vi "singleStamp.vi"() -> ()   [LabVIEW 2017]
uses:
  Gantry/Shared Components/Gantry Class/Type Definitions/Virtual Modes.ctl
  Gantry/Shared Components/Gantry Class/Gantry.lvclass
  Gantry/Shared Components/FlexWorktable/FlexWorktable.lvclass
panel:
  out "error out":errorcluster
  in  "Config Folder":path=path "C:/Users/husker/Desktop/gantry/Config"
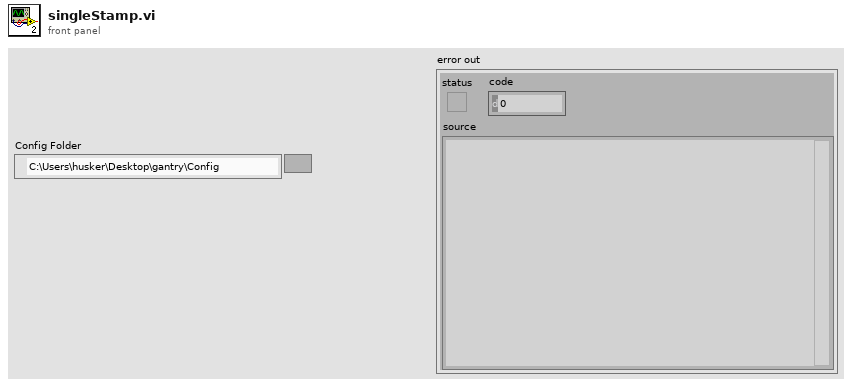
[diagram p1: front panel]
types:
  T1 = typedef "Virtual Modes.ctl" = enum16{"Nonvirtual", "Virtual"}
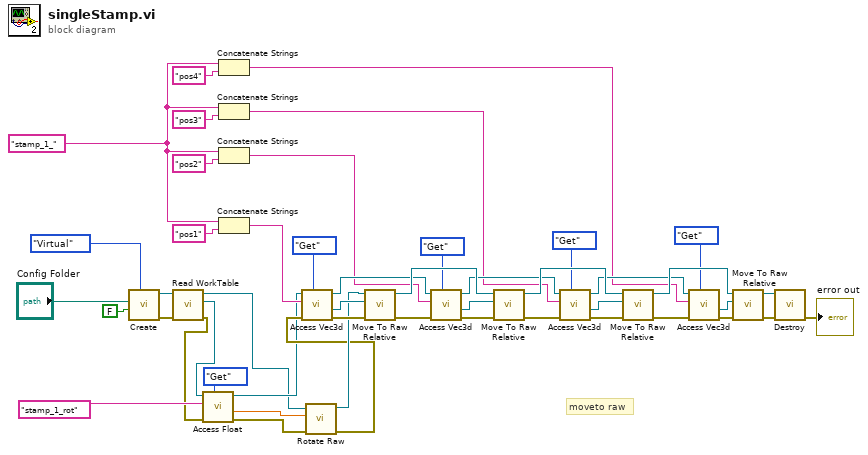
[diagram p0: block diagram]
diagram:
  w17 = "stamp_1_"
  # "moveto raw"
  n1 = call "Create.vi"("Virtual Mode"=Virtual_Modes."Virtual", "HOME?"=FALSE, "Config Folder"="Config Folder") -> ("error out"=w43:errorcluster, "Gantry out"=w44:refnum<class "Gantry.lvclass">)  [unwired: 6 in, 1 out]
  n2 = call-dynamic "Read WorkTable.vi"("error in"=w43, "Gantry Class in"=w44) -> ("error out"=w8:errorcluster, "Worktable"=w9:refnum<class "FlexWorktable.lvclass">, "Gantry Class out"=w2:refnum<class "Gantry.lvclass">)  [unwired: 7 in]
  n3 = call-dynamic "Access Float.vi"("Get/Set"=enum16{"Get", "Set"}."Get", "error in (no error)"=w8, "Key"="stamp_1_rot", "FlexWorktable in"=w9) -> ("error out"=w6:errorcluster, "Value out"=w4:dbl, "FlexWorktable out"=w3:refnum<class "FlexWorktable.lvclass">)  [unwired: 5 in]
  n4 = Concatenate Strings(w17, "pos4" ("string")) -> (w21:string)
  n5 = Concatenate Strings(w17, "pos3" ("string")) -> (w23:string)
  n6 = Concatenate Strings(w17, "pos2" ("string")) -> (w24:string)
  n7 = Concatenate Strings(w17, "pos1" ("string")) -> (w19:string)
  n8 = call-dynamic "Rotate Raw.vi"("error in"=w6, "position(deg)"=w4, "Gantry in"=w2) -> ("error out"=w5:errorcluster, "Gantry out"=w7:refnum<class "Gantry.lvclass">)  [unwired: 7 in]
  n9 = call-dynamic "Access Vec3d.vi"("Get/Set"=enum16{"Get", "Set"}."Get", "error in (no error)"=w5, "Key"=w19, "FlexWorktable in"=w3) -> ("error out"=w14:errorcluster, "Value out"=w41:refnum<class "Vec3d.lvclass">, "FlexWorktable out"=w28:refnum<class "FlexWorktable.lvclass">)  [unwired: 5 in]
  n10 = call-dynamic "Move To Raw Relative.vi"("error in"=w14, "Delta"=w41, "Gantry in"=w7) -> ("error out"=w29:errorcluster, "Gantry out"=w34:refnum<class "Gantry.lvclass">)  [unwired: 7 in]
  n11 = call-dynamic "Access Vec3d.vi"("Get/Set"=enum16{"Get", "Set"}."Get", "error in (no error)"=w29, "Key"=w24, "FlexWorktable in"=w28) -> ("error out"=w40:errorcluster, "Value out"=w39:refnum<class "Vec3d.lvclass">, "FlexWorktable out"=w27:refnum<class "FlexWorktable.lvclass">)  [unwired: 5 in]
  n12 = call-dynamic "Move To Raw Relative.vi"("error in"=w40, "Delta"=w39, "Gantry in"=w34) -> ("error out"=w32:errorcluster, "Gantry out"=w33:refnum<class "Gantry.lvclass">)  [unwired: 7 in]
  n13 = call-dynamic "Access Vec3d.vi"("Get/Set"=enum16{"Get", "Set"}."Get", "error in (no error)"=w32, "Key"=w23, "FlexWorktable in"=w27) -> ("error out"=w38:errorcluster, "Value out"=w37:refnum<class "Vec3d.lvclass">, "FlexWorktable out"=w26:refnum<class "FlexWorktable.lvclass">)  [unwired: 5 in]
  n14 = call-dynamic "Move To Raw Relative.vi"("error in"=w38, "Delta"=w37, "Gantry in"=w33) -> ("error out"=w30:errorcluster, "Gantry out"=w31:refnum<class "Gantry.lvclass">)  [unwired: 7 in]
  n15 = call-dynamic "Access Vec3d.vi"("Get/Set"=enum16{"Get", "Set"}."Get", "error in (no error)"=w30, "Key"=w21, "FlexWorktable in"=w26) -> ("error out"=w36:errorcluster, "Value out"=w35:refnum<class "Vec3d.lvclass">)  [unwired: 5 in, 1 out]
  n16 = call-dynamic "Move To Raw Relative.vi"("error in"=w36, "Delta"=w35, "Gantry in"=w31) -> ("error out"=w15:errorcluster, "Gantry out"=w16:refnum<class "Gantry.lvclass">)  [unwired: 7 in]
  n17 = call "Destroy.vi"("error in"=w15, "Gantry Class in"=w16) -> ("error out"=→"error out":errorcluster)  [unwired: 9 in]
